vi "Vel2Accel.vi"(10 "Acceleration Max":dbl, 11 "Velocities":cluster{"Time":dbl, "Velocity":dbl, "X":dbl}[](array[cluster])) -> (3 "AccelParams":T1(array[cluster]))   [LabVIEW 2014]
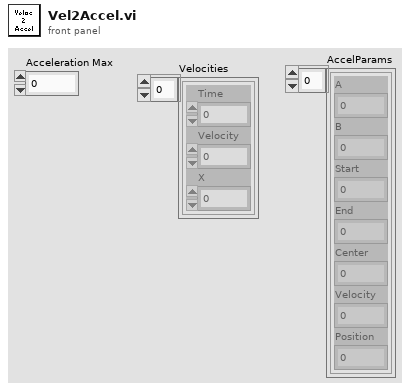
[diagram p1: front panel]
types:
  T1 = cluster{"A":dbl, "B":dbl, "Start":dbl, "End":dbl, "Center":dbl, "Velocity":dbl, "Position":dbl}[]
  T2 = cluster{"A":dbl, "B":dbl, "Start":dbl, "End":dbl, "Center":dbl, "Velocity":dbl, "Position":dbl}
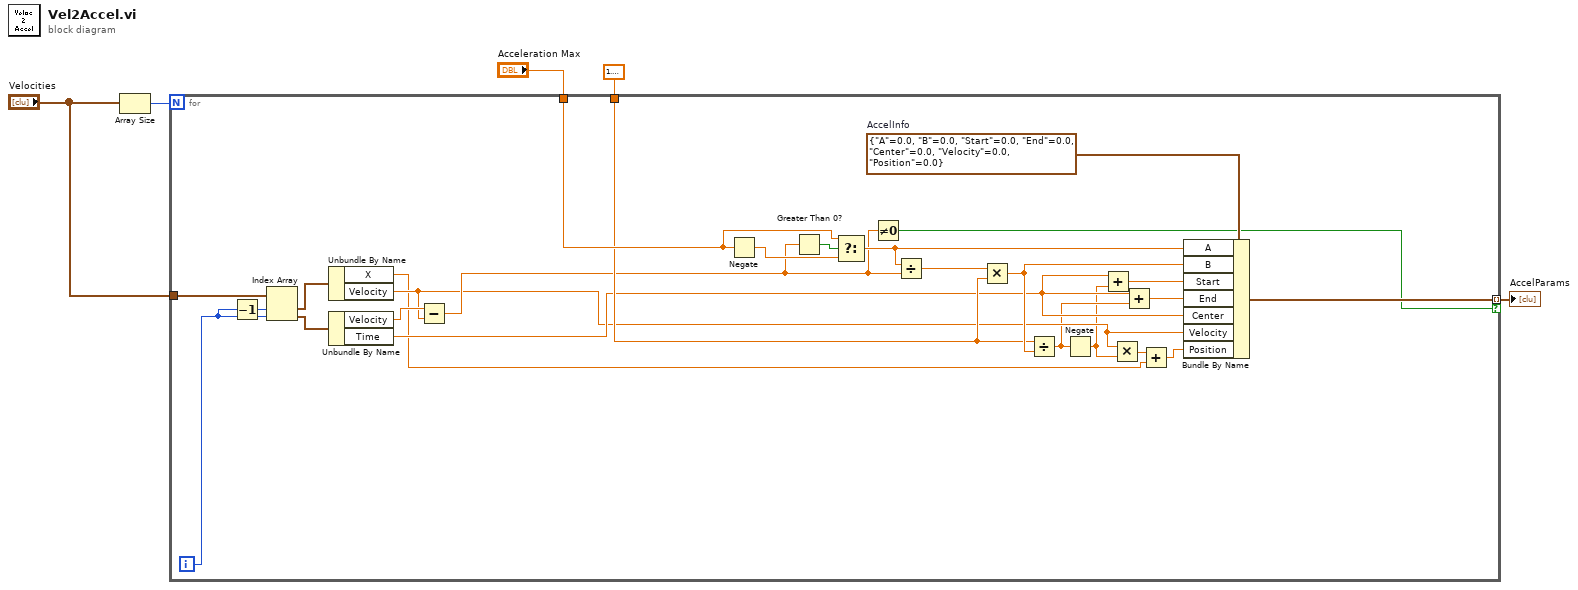
[diagram p0: block diagram]
diagram:
  n1 = Array Size(array="Velocities") -> (size(s)=w5:i32)
  n2 = for {
    N: w5 -> [_]
    tunnel: "Velocities" -> [w27]
    tunnel: "Acceleration Max" -> [w17]
    tunnel: 1.5707963267948966 -> [w16]
    tunnel: [w15] -> w1 mode=indexing if=w12
    i -> [w26]
    w25 = T2 {"A"=0.0, "B"=0.0, "Start"=0.0, "End"=0.0, "Center"=0.0, "Velocity"=0.0, "Position"=0.0}  # AccelInfo
    n3 = Decrement(x=w26) -> (x-1=w28:i32)
    n4 = Index Array(array=w27, index #1=w28, index #2=w26) -> (element #1=w29:cluster{"Time":dbl, "Velocity":dbl, "X":dbl}, element #2=w30:cluster{"Time":dbl, "Velocity":dbl, "X":dbl})
    n5 = Unbundle By Name(w29) -> ("X"=w6:dbl, "Velocity"=w11:dbl)
    n6 = Unbundle By Name(w30) -> ("Velocity"=w31:dbl, "Time"=w14:dbl)
    n7 = Subtract(x=w31, y=w11) -> (x-y=w13:dbl)
    n8 = Negate(x=w17) -> (-x=w24:dbl)
    n9 = Greater Than 0?(x=w13) -> (x > 0?=w23:bool)
    n10 = Select(t=w17, s=w23, f=w24) -> (s? t:f=w22:dbl)
    n11 = Not Equal To 0?(x=w13) -> (x != 0?=w12:bool)
    n12 = Divide(x=w22, y=w13) -> (x/y=w21:dbl)
    n13 = Multiply(x=w21, y=w16) -> (x*y=w18:dbl)
    n14 = Divide(x=w16, y=w18) -> (x/y=w10:dbl)
    n15 = Negate(x=w10) -> (-x=w9:dbl)
    n16 = Add(x=w14, y=w9) -> (x+y=w19:dbl)
    n17 = Multiply(x=w11, y=w9) -> (x*y=w8:dbl)
    n18 = Add(x=w14, y=w10) -> (x+y=w20:dbl)
    n19 = Add(x=w8, y=w6) -> (x+y=w7:dbl)
    n20 = Bundle By Name(cluster=w25, "A"=w22, "B"=w18, "Start"=w19, "End"=w20, "Center"=w14, "Velocity"=w11, "Position"=w7) -> (w15:T2)
  }
  "AccelParams" <- w1
